vi "SERIAL_VerifyTermination.vi"(2 "ExpectedFullPacketLength":i32, 3 "Packet\n\n\n\n\n\n\n\n\n\n\n\n\n\nPacketContent":string) -> (0 "OffsetPastTermination":i32, 1 "ValidTermination":bool)   [LabVIEW 2014, in "navX-MXP IMU.lvlib"]
uses:
  navX-MXP IMU.lvlib
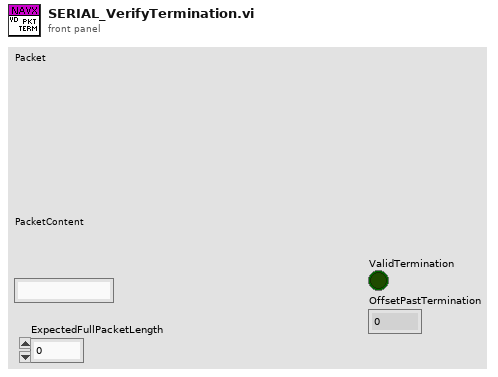
[diagram p1: front panel]
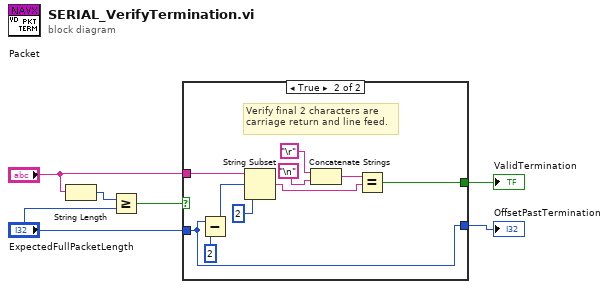
[diagram p0: block diagram]
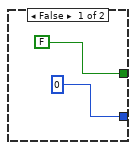
[diagram p2: hidden frame]
diagram:
  n1 = String Length(string="Packet\n\n\n\n\n\n\n\n\n\n\n\n\n\nPacketContent") -> (length=w4:i32)
  n2 = Greater Or Equal?(x=w4, y="ExpectedFullPacketLength") -> (x >= y?=w3:bool)
  n3 = case shown="True" w3 {
    tunnel: "Packet\n\n\n\n\n\n\n\n\n\n\n\n\n\nPacketContent" -> [_ w18]
    tunnel: [FALSE w12] -> w5
    tunnel: [0 w10] -> w2
    tunnel: "ExpectedFullPacketLength" -> [_ w10]
    frame False {
    }
    frame True {
      # "Verify final 2 characters are \ncarriage return and line feed."
      n4 = Subtract(x=w10, y=2) -> (x-y=w9:i32)
      n5 = String Subset(string=w18, offset (0)=w9, length (rest)=2 ("y")) -> (substring=w13:string)
      n6 = Concatenate Strings("\r", "\n") -> (w14:string)
      n7 = Equal?(x=w14, y=w13) -> (x = y?=w12:bool)
    }
  }
  "ValidTermination" <- w5
  "OffsetPastTermination" <- w2
